vi "Day 16-1.vi"() -> ()   [LabVIEW 2019, in "Day 16.lvlib"]
uses:
  Day 16.lvlib
  Controls/Packet.ctl
panel:
  out "sum":u32
  out "Packets Out":T1[](array[typedef])
  out "Bit Stream":bool[](array[boolean])
  in  "String":string="E20D72805F354AE298E2FCC5339218F90FE5F3A388BA60095005C3352CF7FBF27CD4B3DFEFC95354723006C401C8FD1A23280021D1763CC791006E25C198A6C01254BAECDED7A5A99CCD30C01499CFB948F857002BB9FCD68B3296AF23DD6BE4C600A4D3ED006AA200C4128E10FC0010C8A90462442A5006A7EB2429F8C502675D13700BE37CF623EB3449CAE732249279EFDED801E898A47BE8D23FBAC0805527F99849C57A5270C064C3ECF577F4940016A269007D3299D34E004DF298EC71ACE8DA7B77371003A76531F20020E5C4CC01192B3FE80293B7CD23ED55AA76F9A47DAAB6900503367D240522313ACB26B8801B64CDB1FB683A6E50E0049BE4F6588804459984E98F28D80253798DFDAF4FE712D679816401594EAA580232B19F20D92E7F3740D1003880C1B0..."
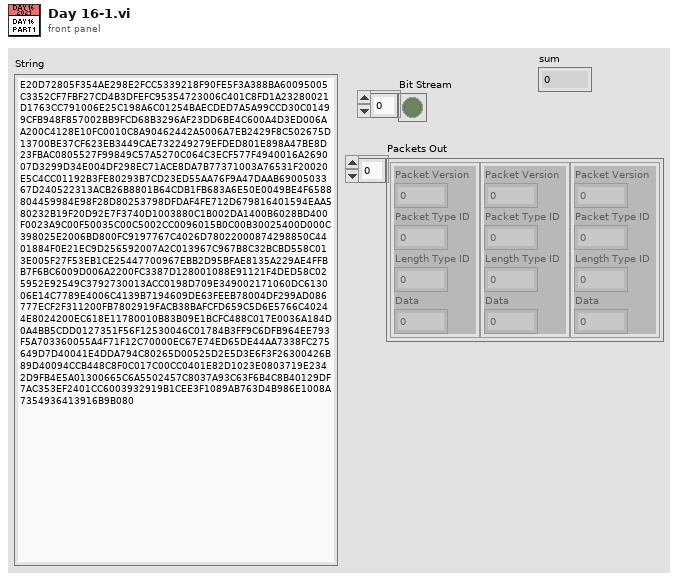
[diagram p1: front panel]
types:
  T1 = typedef "Day 16.lvlib/Packet.ctl" = cluster{"Packet Version":u32, "Packet Type ID":u32, "Length Type ID":u32, "Data":u64}
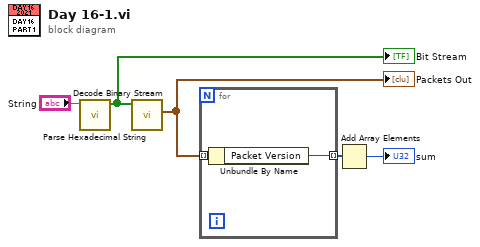
[diagram p0: block diagram]
diagram:
  n1 = call "Parse Hexadecimal String.vi"("Hex String"="String") -> ("Bit Stream"=w4:bool[])  [unwired: 10 in]
  "Bit Stream" <- w4
  n2 = call "Decode Binary Stream.vi"("Bit Stream"=w4) -> ("Packets Out"=w3:T1[])  [unwired: 9 in, 1 out]
  "Packets Out" <- w3
  n3 = for {
    tunnel: w3 -> [w7] mode=indexing
    tunnel: [w6] -> w2 mode=indexing
    n4 = Unbundle By Name(w7) -> ("Packet Version"=w6:u32)
  }
  n5 = Add Array Elements(numeric array=w2) -> (sum=→"sum":u32)
